vi "Get CN Enable.vi"(3 "Images":T1[](array[typedef]), 4 "CN Config":T2[](array[typedef]), 5 "filenames":string[](array[string])) -> (1 "CN Config out":T2[](array[typedef]), 2 "image Enable":T1[](array[typedef]))   [LabVIEW 2014]
uses:
  Type'def/CN Config Ctr.ctl
  <vilib>/picture/picture.llb/imagedata.ctl
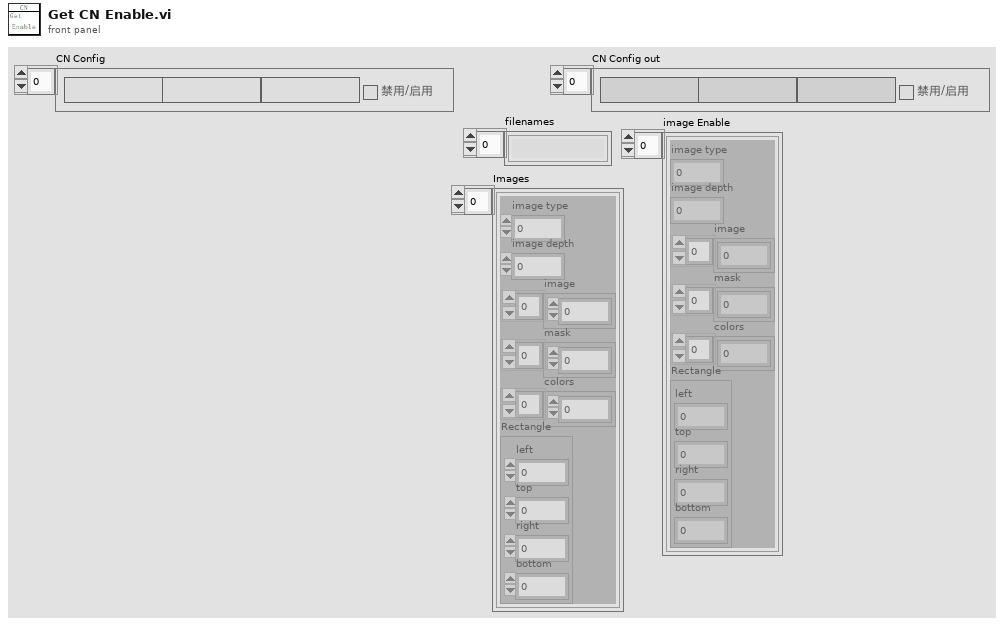
[diagram p1: front panel]
types:
  T1 = typedef "imagedata.ctl" = cluster{"image type":i32, "image depth":i32, "image":u8[], "mask":u8[], "colors":u32[], "Rectangle":cluster{"left":i16, "top":i16, "right":i16, "bottom":i16}}
  T2 = typedef "CN Config Ctr.ctl" = cluster{"Model":string, "Pic_Name":string, "CarName":string, "En/Disable":bool}
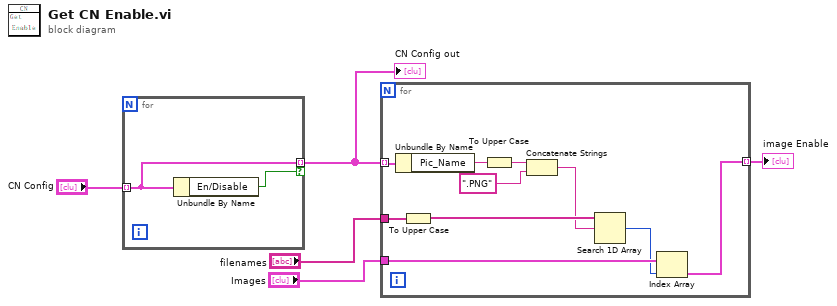
[diagram p0: block diagram]
diagram:
  n1 = for {
    tunnel: "CN Config" -> [w7] mode=indexing
    tunnel: [w7] -> w4 mode=indexing if=w6
    n2 = Unbundle By Name(w7) -> ("En/Disable"=w6:bool)
  }
  "CN Config out" <- w4
  n3 = for {
    tunnel: w4 -> [w17] mode=indexing
    tunnel: "filenames" -> [w16]
    tunnel: "Images" -> [w10]
    tunnel: [w8] -> w1 mode=indexing
    n4 = Unbundle By Name(w17) -> ("Pic_Name"=w15:string)
    n5 = To Upper Case(1:w16) -> (0:w12:string[])
    n6 = To Upper Case(1:w15) -> (0:w14:string)
    n7 = Concatenate Strings(w14, ".PNG") -> (w11:string)
    n8 = Search 1D Array(1D array=w12, element=w11) -> (index of element=w9:i32)  [unwired: 1 in]
    n9 = Index Array(array=w10, index=w9) -> (element=w8:T1)
  }
  "image Enable" <- w1
